vi "Open.vi"(8 "error in (no error)":errorcluster, 11 "Ini File in":refnum<class "Ini File.lvclass">) -> (0 "error out":errorcluster, 3 "Ini File out":refnum<class "Ini File.lvclass">)   [LabVIEW 2021, in "File Library.lvlib" / "Ini File.lvclass"]
uses:
  Ini File.lvclass
  Ini File.lvclass/Ini File.ctl
  <vilib>/Utility/config.llb/NI_LVConfig.lvlib
  User Connections/User Connections.lvclass
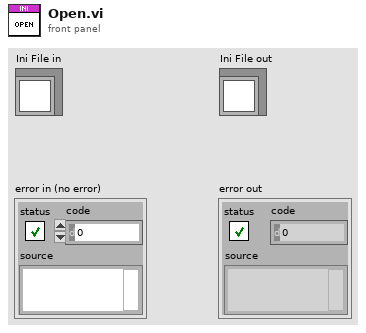
[diagram p1: front panel]
types:
  T1 = typedef "NI_LVConfig.lvlib/Config Data RefNum.ctl" = refnum<k1>
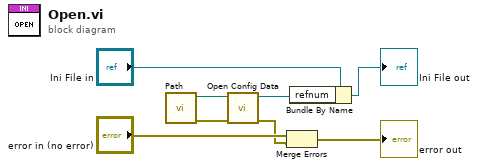
[diagram p0: block diagram]
diagram:
  n1 = call "Path.vi"() -> ("error out"=w1:errorcluster, "Path"=w2:path)  [unwired: 10 in]
  n2 = call <vilib>:"Open Config Data.vi"("error in (no error)"=w1, "configuration file path"=w2) -> ("error out"=w3:errorcluster, "refnum"=w5:T1)  [unwired: 7 in, 1 out]
  n3 = Merge Errors("error in (no error)", w3) -> (→"error out":errorcluster)
  n4 = Bundle By Name(cluster="Ini File in", "refnum"=w5) -> (→"Ini File out":refnum<class "Ini File.lvclass">)
